vi "JSON String.vi"(1 "in":string) -> (0 "out":string)   [LabVIEW 2013, in "LV JSON.lvlib"]
uses:
  LV JSON.lvlib
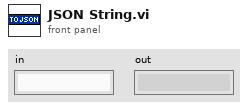
[diagram p1: front panel]
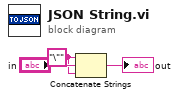
[diagram p0: block diagram]
diagram:
  w2 = "\"" ("string")
  n1 = Concatenate Strings(w2, "in", w2) -> (→"out":string)
